vi "Copy_Settings.vi"(8 "error in (no error)":errorcluster, 10 "LabVIEW Object":refnum<class>, 11 "IB_Settings_Item_File in":refnum<class "IB_Settings_Item_File.lvclass">) -> (0 "error out":errorcluster, 3 "IB_Settings_Item_File out":refnum<class "IB_Settings_Item_File.lvclass">)   [LabVIEW 2020, in "IB_Settings_Item_File.lvclass"]
uses:
  <vilib>/AppBuilder/IB_Classes/Settings_Item_File/IB_Settings_Item_File.lvclass
  <vilib>/AppBuilder/IB_Classes/Settings_Item_File/IB_Settings_Item_File.lvclass/IB_Settings_Item_File.ctl
  <vilib>/AppBuilder/IB_Classes/Source/File/IB_Source_File.lvclass
  <vilib>/AppBuilder/IB_Classes/Settings_Item/IB_Settings_Item.lvclass
  <vilib>/AppBuilder/IB_Classes/Source/IB_Source.lvclass
  e:/builds/penguin/labview/branches/2020/dev/dist/vi.lib/AppBuilder/IB_Classes/Settings_Item/IB_Settings_Item.lvclass
  e:/builds/penguin/labview/branches/2020/dev/dist/vi.lib/AppBuilder/IB_Classes/Settings_Item_File/IB_Settings_Item_File.lvclass
  e:/builds/penguin/labview/branches/2020/dev/dist/vi.lib/AppBuilder/IB_Classes/Source/IB_Source.lvclass
  e:/builds/penguin/labview/branches/2020/dev/dist/vi.lib/AppBuilder/IB_Classes/Source/File/IB_Source_File.lvclass
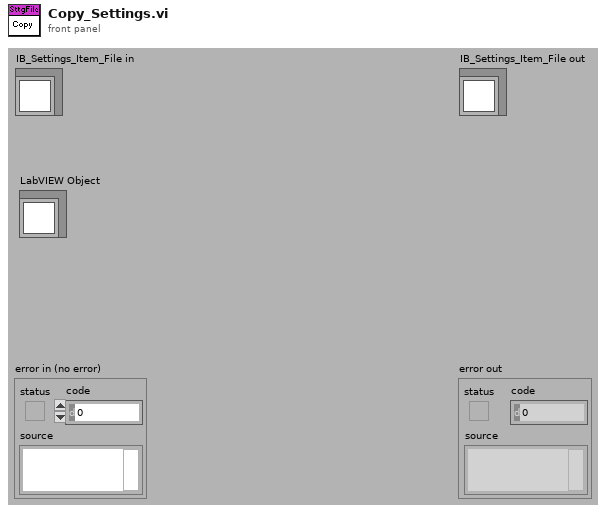
[diagram p1: front panel]
types:
  T1 = typedef "IB_Source.ctl" = cluster{"name":string, "sourceTag":string, "destTag":string, "path":path, "eng_installPath":string, "UI_inBuild?":bool, "str ref?":bool}
  T2 = typedef "IB_Source_File.ctl" = cluster{"Attributes":i16, "RegCOM":bool, "unlock":bool, "shortcuts":refnum<class "IB_Shortcut.lvclass">[], "EXE_install":bool, "CmdArg_install":string, "EXE_uninstall":bool, "CmdArg_uninstall":string}
  T3 = typedef "IB_Settings_Item.ctl" = cluster{"address":string[], "Attributes":i16, "RegCOM":bool, "unlock":bool}
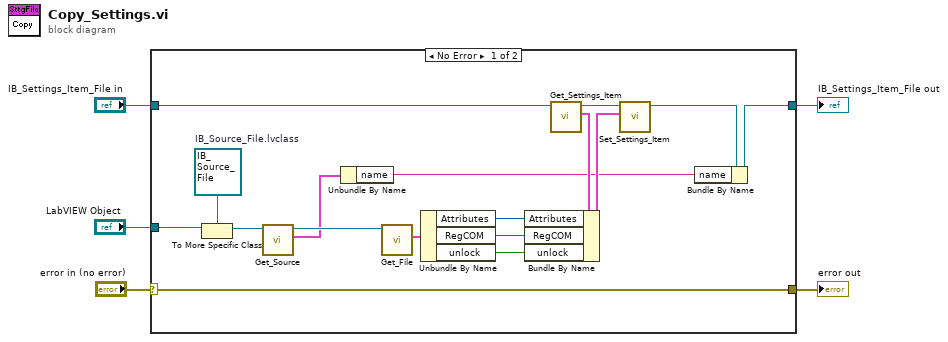
[diagram p0: block diagram]
diagram:
  n1 = case shown="No Error" "error in (no error)" {
    selector: "error in (no error)" -> [w6 w24]
    tunnel: "LabVIEW Object" -> [w22 _]
    tunnel: [w6 w24] -> w3
    tunnel: "IB_Settings_Item_File in" -> [w19 w23]
    tunnel: [w9 w23] -> w1
    frame No Error {
      w21 = refnum<class "IB_Source_File.lvclass"> refnum  # IB_Source_File.lvclass
      n2 = To More Specific Class(target class=w21, reference=w22) -> (specific class reference=w12:refnum<class "IB_Source_File.lvclass">)  [unwired: 1 in, 1 out]
      n3 = call <vilib>:"Get_Source.vi"("IB_Source in"=w12) -> ("data"=w8:T1, "IB_Source out"=w11:refnum<class "IB_Source_File.lvclass">)  [unwired: 1 in, 8 out]
      n4 = Unbundle By Name(w8) -> ("name"=w7:string)
      n5 = call <vilib>:"Get_File.vi"("IB_Source_File in"=w11) -> ("data"=w20:T2)  [unwired: 1 in, 9 out]
      n6 = Unbundle By Name(w20) -> ("Attributes"=w15:i16, "RegCOM"=w14:bool, "unlock"=w13:bool)
      n7 = call <vilib>:"Get_Settings_Item.vi"("IB_Settings_Item in"=w19) -> ("data"=w17:T3, "IB_Settings_Item out"=w18:refnum<class "IB_Settings_Item_File.lvclass">)  [unwired: 1 in, 8 out]
      n8 = Bundle By Name(cluster=w17, "Attributes"=w15, "RegCOM"=w14, "unlock"=w13) -> (w16:T3)
      n9 = call <vilib>:"Set_Settings_Item.vi"("data"=w16, "IB_Settings_Item in"=w18) -> ("IB_Settings_Item out"=w10:refnum<class "IB_Settings_Item_File.lvclass">)  [unwired: 1 in, 8 out]
      n10 = Bundle By Name(cluster=w10, "name"=w7) -> (w9:refnum<class "IB_Settings_Item_File.lvclass">)
    }
    frame Error {
    }
  }
  "error out" <- w3
  "IB_Settings_Item_File out" <- w1
